vi "call.vi"(8 "error in (no error)":errorcluster, 10 "Parameters in":refnum<class "IBaseObject.lvclass">, 11 "IFunction in":refnum<class "IFunction.lvclass">) -> (0 "error out":errorcluster, 1 "Result out":refnum<class "IBaseObject.lvclass">, 2 "Parameters out":refnum<class "IBaseObject.lvclass">, 3 "IFunction out":refnum<class "IFunction.lvclass">)   [LabVIEW 2022 SP3, in "openDAQ.lvlib" / "daqCoreTypes.lvlib" / "IFunction.lvclass"]
uses:
  <instrlib>/openDAQ/Public/Classes/daqCoreTypes/IFunction/IFunction.lvclass
  <instrlib>/openDAQ/Public/Classes/daqCoreTypes/IFunction/IFunction.lvclass/IFunction.ctl
  <instrlib>/openDAQ/Binaries/Windows/x86/copendaq32.dll
  <instrlib>/openDAQ/Public/Classes/IBaseObject/IBaseObject.lvclass
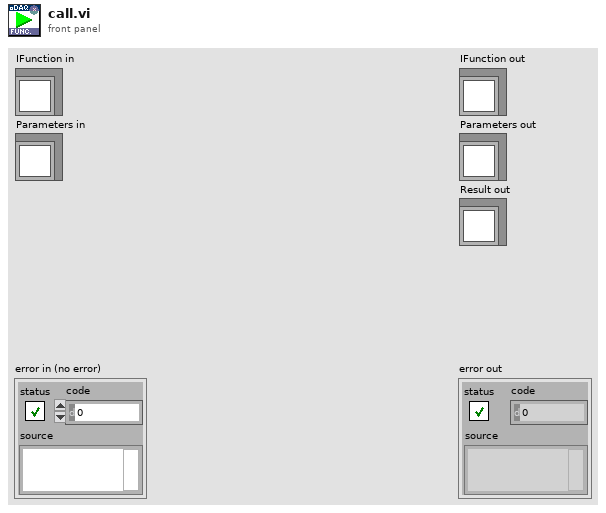
[diagram p1: front panel]
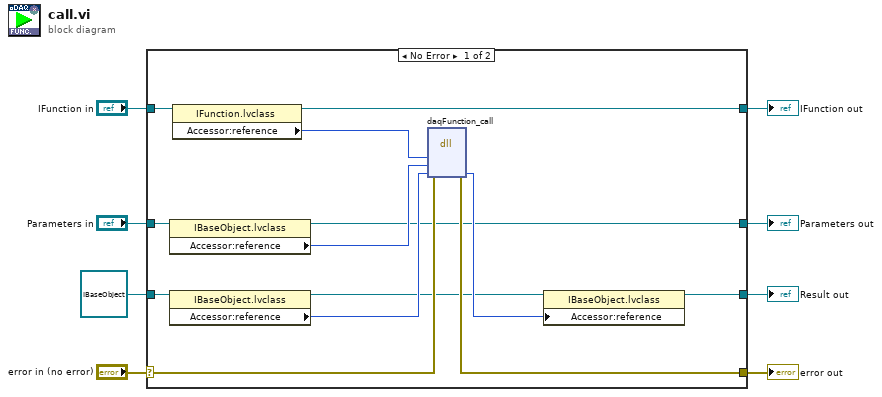
[diagram p0: block diagram]
diagram:
  n1 = case shown="No Error" "error in (no error)" {
    selector: "error in (no error)" -> [w20 w25]
    tunnel: [w19 w25] -> w7
    tunnel: [w18 w24] -> w5
    tunnel: "IFunction in" -> [w21 w24]
    tunnel: "Parameters in" -> [w16 w23]
    tunnel: [w10 w23] -> w3
    tunnel: refnum<class "IBaseObject.lvclass"> refnum ("openDAQ.lvlib:IBaseObject.lvlib:IBaseObject.lvclass") -> [w14 w22]
    tunnel: [w9 w22] -> w1
    frame No Error {
      n2 = property class="IBaseObject.lvclass"(reference=w16) -> (reference out=w10:refnum<class "IBaseObject.lvclass">, "Accessor:reference"=w15:i64)  [unwired: 1 in, 1 out]
      n3 = property class="IBaseObject.lvclass"(reference=w14) -> (reference out=w11:refnum<class "IBaseObject.lvclass">, "Accessor:reference"=w13:i64)  [unwired: 1 in, 1 out]
      n4 = property class="IFunction.lvclass"(reference=w21) -> (reference out=w18:refnum<class "IFunction.lvclass">, "Accessor:reference"=w17:i64)  [unwired: 1 in, 1 out]
      n5 = dll-call lib="C:/Program Files (x86)/National Instruments/LabVIEW 2022/instr.lib/openDAQ/Binaries/Windows/x86/copendaq*.*" fn="daqFunction_call"(error in=w20, "function"=w17, "params"=w15, "result"=w13) -> (error out=w19:errorcluster, "result"=w12:i64)  [unwired: 5 in, 1 out]
      n6 = property class="IBaseObject.lvclass"(reference=w11, "Accessor:reference"=w12) -> (reference out=w9:refnum<class "IBaseObject.lvclass">)  [unwired: 1 in, 1 out]
    }
    frame Error {
    }
  }
  "error out" <- w7
  "IFunction out" <- w5
  "Parameters out" <- w3
  "Result out" <- w1
